vi "Create.vi"(8 "error in (no error)":errorcluster) -> (0 "error out":errorcluster, 3 "SimTask out":refnum<class "SimTask.lvclass">)   [LabVIEW 2020, in "VolatusDemo.lvlib" / "SimTask.lvclass"]
uses:
  SimTask.lvclass
  SimTask.lvclass/SimTask.ctl
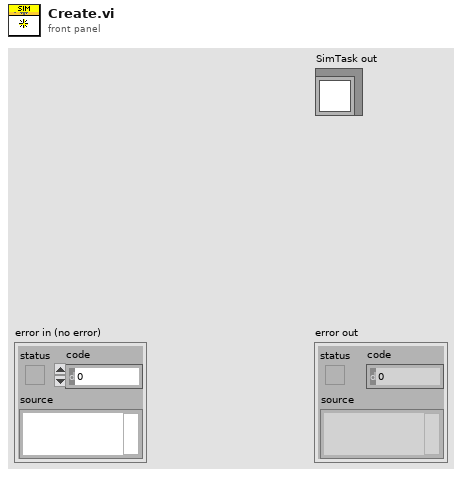
[diagram p1: front panel]
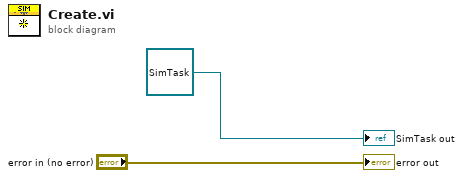
[diagram p0: block diagram]
diagram:
  "error out" <- "error in (no error)"
  "SimTask out" <- refnum<class "SimTask.lvclass"> refnum ("SimTask in")
